vi "PowerSupply.vi"() -> ()   [LabVIEW 2018]
uses:
  classes/Tushars Events Toolkit/Software/Modules/EventClient_ObjectReference.ctl
  classes/Variable Manager/VariableManager_Bool.vi
  Strict Type Controls/Settings Operation.ctl
  ThirdParty/Keithley KE22xx Series/Keithley KE22xx Series.lvlib
  ThirdParty/Agilent E364X Series/Agilent E364X Series.lvlib
  classes/Variable Manager/VariableManager_Double.vi
panel:
  out "Quit":bool
  out "error out":errorcluster
  in  "error in (no error)":errorcluster
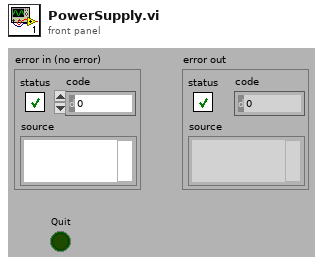
[diagram p1: front panel]
types:
  T1 = cluster{"Port":refnum<visa-resource-name>, "baud rate":u32, "data bits":u16, "parity":enum16{"None", "Odd", "Even", "Mark", "Space"}, "stop bits":u16, "flow control":u16, "timeout":u32}
  T2 = cluster{"PSPort":refnum<visa-resource-name>, "lastUpdate":u32}
  T3 = typedef "EventClient_ObjectReference.ctl" = refnum<k1>
  T4 = typedef "Settings Operation.ctl" = enum8{"Get Value", "Set Value", "Read File", "Write File", "Write Stored Value"}
  T5 = cluster{"Port":refnum<visa-resource-name>, "baud rate":u32, "data bits":u16, "stop bits":u16, "parity":enum16{"None", "Odd", "Even", "Mark", "Space"}, "flow control":u16, "Timeout":u32}
  T6 = cluster{"Instrument Select (Output 1)":string, dbl}
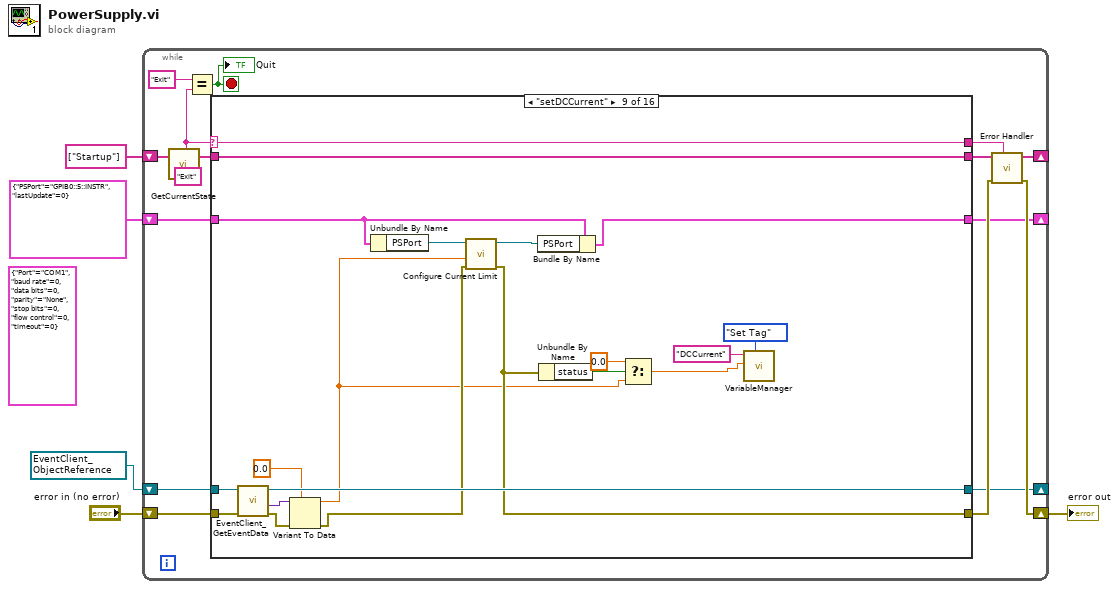
[diagram p0: block diagram]
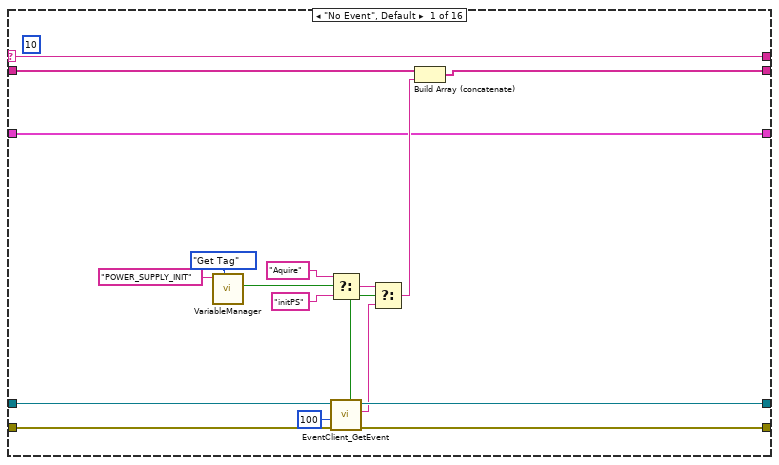
[diagram p2: hidden frame]
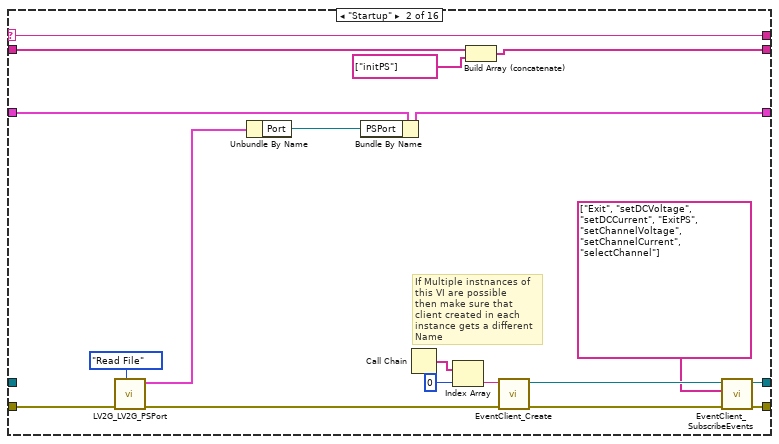
[diagram p3: hidden frame]
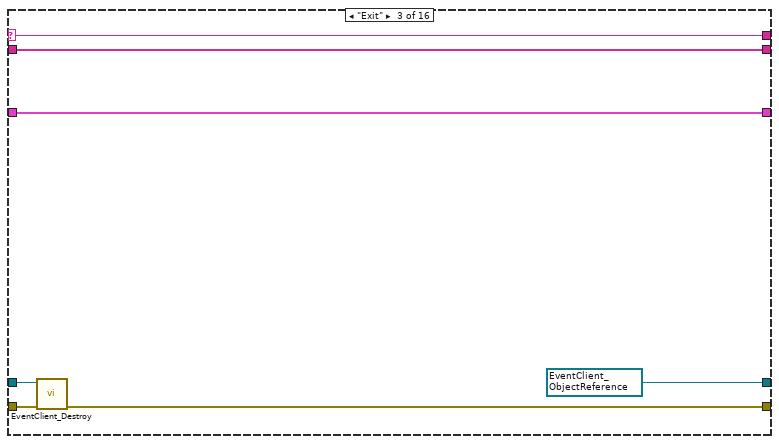
[diagram p4: hidden frame]
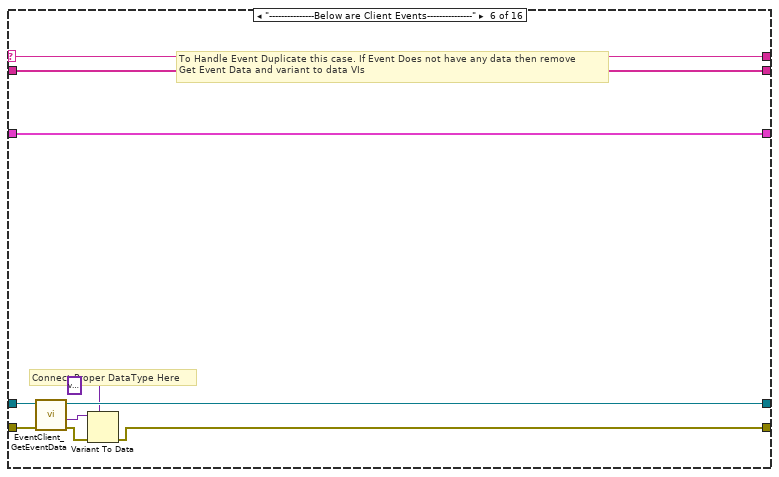
[diagram p7: hidden frame]
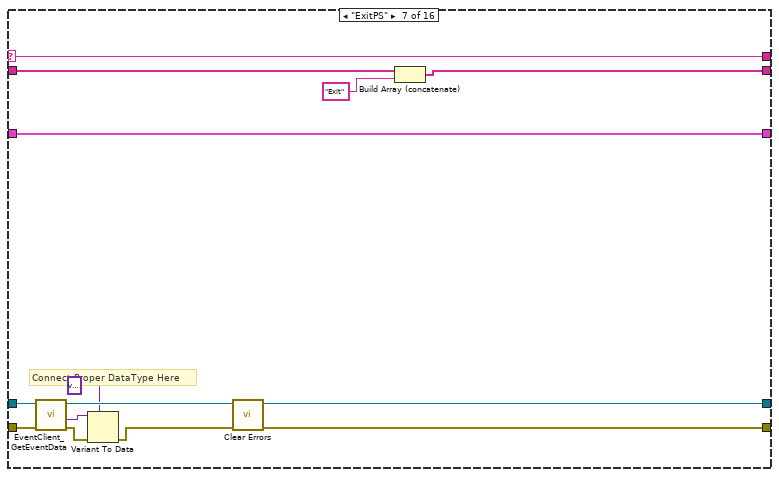
[diagram p8: hidden frame]
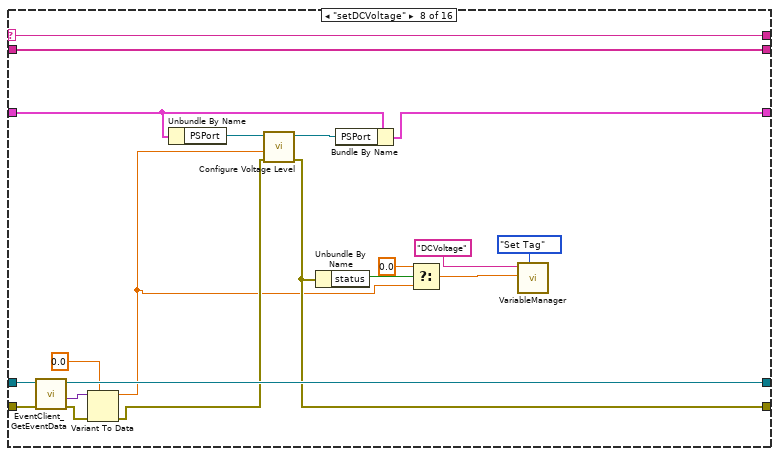
[diagram p9: hidden frame]
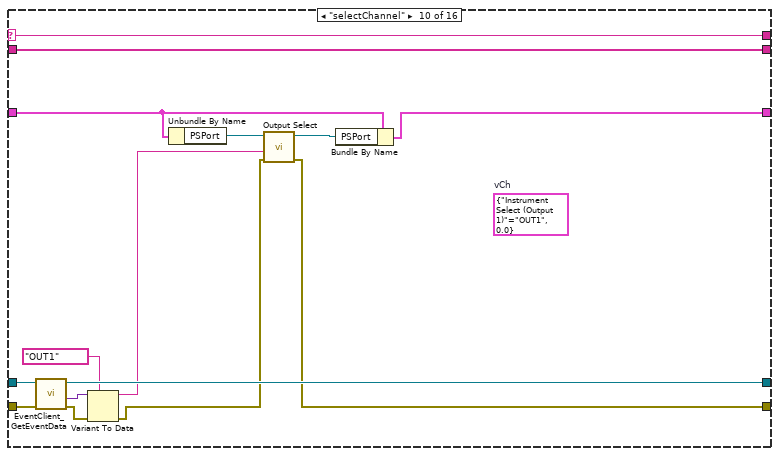
[diagram p10: hidden frame]
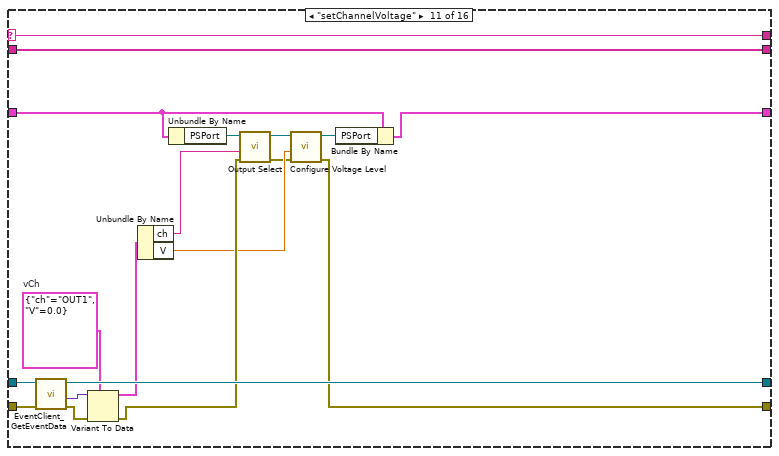
[diagram p11: hidden frame]
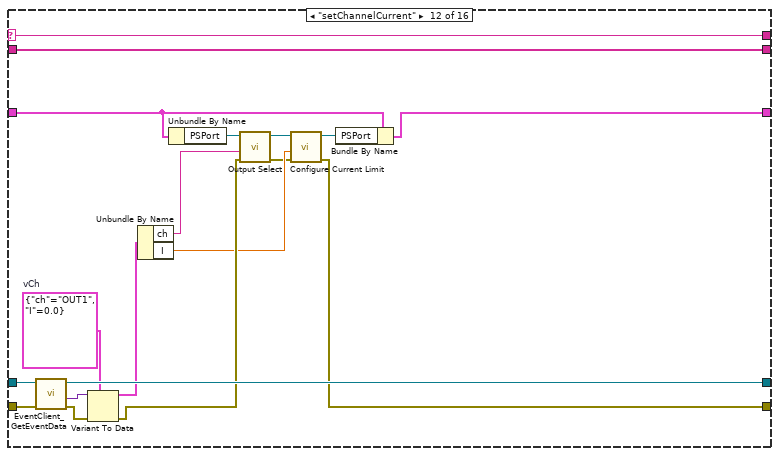
[diagram p12: hidden frame]
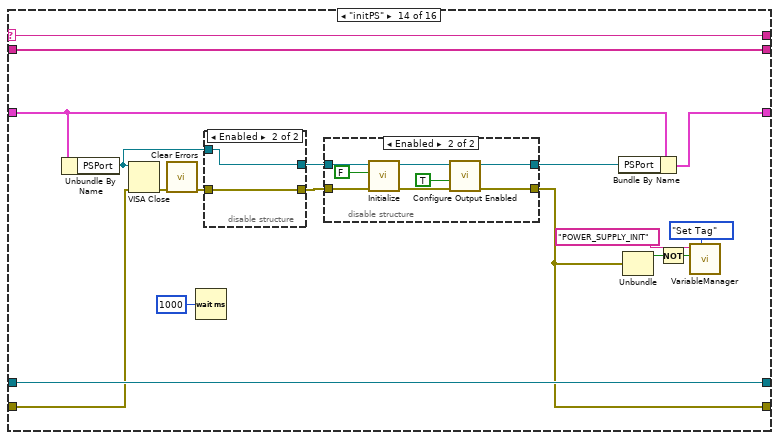
[diagram p14: hidden frame]
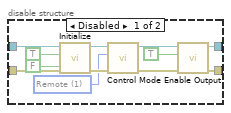
[diagram p15: hidden frame]
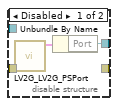
[diagram p16: hidden frame]
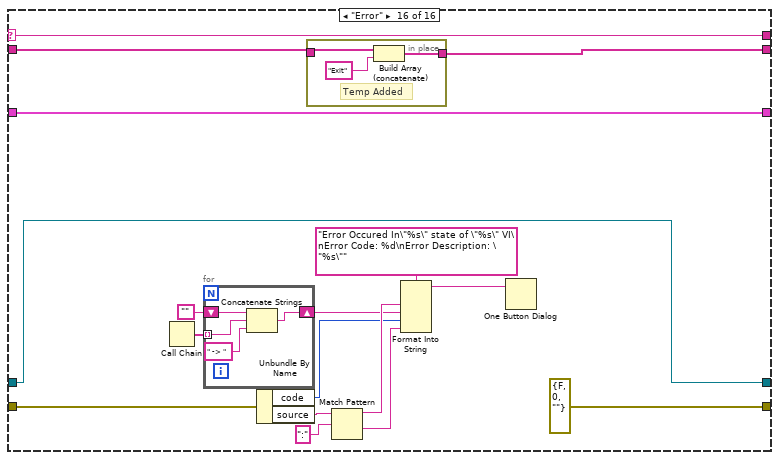
[diagram p18: hidden frame]
diagram:
  (unwired) T1 {"Port"="COM1", "baud rate"=0, "data bits"=0, "parity"=enum."None", "stop bits"=0, "flow control"=0, "timeout"=0} ("Merlin")
  w2 = T3 refnum items=["EventClient"] ("reference")
  n1 = while {
    shift-right: [w16] -> _
    shift-left: string[] ["Startup"] ("State Array Out") -> [w20]
    shift-right: [w12] -> w3
    shift-left: "error in (no error)" -> [w13]
    shift-right: [w9] -> _
    shift-left: w2 -> [w8]
    shift-right: [w6] -> _
    shift-left: T2 {"PSPort"="GPIB0::5::INSTR", "lastUpdate"=0} -> [w7]
    stop <- w17 stop-if-true
    (unwired) "Exit" ("x")
    n2 = call "GetCurrentState.vi"("State Array In"=w20) -> ("Current State"=w10:string, "State Array Out"=w19:string[])  [unwired: 17 in]
    n3 = Equal?(x="Exit", y=w10) -> (x = y?=w17:bool)
    "Quit" <- w17
    n4 = case shown="\"setDCCurrent\"" w10 {
      selector: w10 -> [w38 w57 w64 w68 w73 w83 w96 w116 w136 w151 w170 w189 w194 w212 w243 w260]
      tunnel: w19 -> [w31 w56 w63 w69 w74 w84 w97 w117 w137 w152 w171 w190 w195 w213 w242 w247]
      tunnel: [w33 w55 w63 w69 w74 w84 w88 w117 w137 w152 w171 w190 w195 w213 w242 w244] -> w15
      tunnel: [w35 w49 w60 w67 w72 w79 w85 w103 w122 w141 w153 w172 w193 w199 w241 errorcluster {"status"=FALSE, "code"=0, "source"=""} ("error in (no error)")] -> w11
      tunnel: [w38 w57 w64 w68 w73 w83 w96 w116 w136 w151 w170 w189 w194 w212 w243 w260] -> w14
      tunnel: w13 -> [w36 w44 w61 w67 w72 w81 w94 w114 w134 w149 w168 w187 w193 w197 w241 w248]
      tunnel: [w34 w47 w59 w66 w71 w77 w90 w111 w131 w146 w165 w184 w192 w211 w240 w246] -> w9
      tunnel: w8 -> [w37 _ w62 w66 w71 w82 w95 w115 w135 w150 w169 w188 w192 w211 w240 w246]
      tunnel: w7 -> [w24 w45 w58 w65 w70 w75 w86 w109 w129 w145 w164 w183 w191 w204 w239 w245]
      tunnel: [w24 w40 w58 w65 w70 w75 w86 w108 w128 w144 w163 w182 w191 w203 w239 w245] -> w6
      frame "No Event", Default {
        (unwired) 10
        n5 = call-poly "VariableManager.vi"("Operation"=enum16{"Get Tag", "Set Tag"}."Get Tag", "Tag"="POWER_SUPPLY_INIT") -> ("Value out"=w21:bool)  [unwired: 6 in, 3 out]
        n6 = Select(t="Aquire" ("x"), s=w21, f="initPS" ("x")) -> (s? t:f=w26:string)
        n7 = call "EventClient_GetEvent.vi"("error in (no error)"=w36, "timeout in ms (-1)"=100, "reference"=w37) -> ("error out"=w35:errorcluster, "Name"=w29:string, "reference out"=w34:T3, "timed out?"=w30:bool)  [unwired: 4 in, 1 out]
        n8 = Select(t=w26, s=w30, f=w29) -> (s? t:f=w25:string)
        n9 = Build Array (concatenate)(w31, w25) -> (w33:string[])
      }
      frame "Startup" {
        # "If Multiple instnances of this VI are possible \nthen make sure that client created in each instance gets a different Name"
        n10 = call "LV2G_LV2G_PSPort.vi"("Operation"=Settings_Operation."Read File", "error in (no error)"=w44) -> ("error out"=w43:errorcluster, "Modbus485 Out"=w41:T5)  [unwired: 8 in]
        n11 = Unbundle By Name(w41) -> ("Port"=w39:refnum<visa-resource-name>)
        n12 = Bundle By Name(cluster=w45, "PSPort"=w39) -> (w40:T2)
        n13 = Call Chain() -> (call chain=w53:string[])
        n14 = Index Array(array=w53, index=0) -> (element=w51:string)
        n15 = Build Array (concatenate)(w56, string[] ["initPS"] ("State Array Out")) -> (w55:string[])
        n16 = call "EventClient_Create.vi"("error in (no error)"=w43, "Instance Name"=w51) -> ("error out"=w50:errorcluster, "reference"=w48:T3)  [unwired: 8 in]
        n17 = call "EventClient_SubscribeEvents.vi"("error in (no error)"=w50, "Events"=string[] ["Exit", "setDCVoltage", "setDCCurrent", "ExitPS", "setChannelVoltage", "setChannelCurrent", "selectChannel"], "reference"=w48) -> ("error out"=w49:errorcluster, "reference out"=w47:T3)  [unwired: 7 in]
      }
      frame "Exit" {
        w59 = T3 refnum items=["EventClient"] ("reference out")
        n18 = call "EventClient_Destroy.vi"("error in (no error)"=w61, "reference"=w62) -> ("error out"=w60:errorcluster)  [unwired: 9 in]
      }
      frame "---------------Below are UI Events---------------" {
        # "This State will never Execute\nIt is added just for improving code readability please do not remove this case"
      }
      frame "---------------Below are Menu Events---------------" {
        # "This State will never Execute\nIt is added just for improving code readability please do not remove this case"
      }
      frame "---------------Below are Client Events---------------" {
        # "To Handle Event Duplicate this case. If Event Does not have any data then remove\nGet Event Data and variant to data VIs"
        # "Connect Proper DataType Here"
        n19 = call "EventClient_GetEventData.vi"("error in (no error)"=w81, "reference"=w82) -> ("error out"=w80:errorcluster, "Data"=w78:variant, "reference out"=w77:T3)  [unwired: 7 in]
        n20 = Variant To Data(error in=w80, type=variant, Variant=w78) -> (error out=w79:errorcluster)  [unwired: 1 out]
      }
      frame "ExitPS" {
        # "Connect Proper DataType Here"
        n21 = call "EventClient_GetEventData.vi"("error in (no error)"=w94, "reference"=w95) -> ("error out"=w93:errorcluster, "Data"=w91:variant, "reference out"=w90:T3)  [unwired: 7 in]
        n22 = Variant To Data(error in=w93, type=variant, Variant=w91) -> (error out=w92:errorcluster)  [unwired: 1 out]
        n23 = call <vilib>:"Clear Errors.vi"("error in (no error)"=w92) -> ("error out"=w85:errorcluster)  [unwired: 5 in, 1 out]
        n24 = Build Array (concatenate)(w97, "Exit" ("x")) -> (w88:string[])
      }
      frame "setDCVoltage" {
        n25 = call "EventClient_GetEventData.vi"("error in (no error)"=w114, "reference"=w115) -> ("error out"=w113:errorcluster, "Data"=w112:variant, "reference out"=w111:T3)  [unwired: 7 in]
        n26 = Variant To Data(error in=w113, type=0.0, Variant=w112) -> (data=w100:dbl, error out=w106:errorcluster)
        n27 = Unbundle By Name(w109) -> ("PSPort"=w105:refnum<visa-resource-name>)
        n28 = call "Configure Voltage Level.vi"("error in (no error)"=w106, "Level (0.0 Volts)"=w100, "VISA resource name"=w105) -> ("error out"=w103:errorcluster, "VISA resource name out"=w107:refnum<visa-resource-name>)  [unwired: 7 in]
        n29 = Unbundle By Name(w103) -> ("status"=w101:bool)
        n30 = Bundle By Name(cluster=w109, "PSPort"=w107) -> (w108:T2)
        n31 = Select(t=0.0, s=w101, f=w100) -> (s? t:f=w99:dbl)
        n32 = call-poly "VariableManager.vi"("Operation"=enum16{"Get Tag", "Set Tag"}."Set Tag", "Value"=w99, "Tag"="DCVoltage") -> ()  [unwired: 4 in, 5 out]
      }
      frame "setDCCurrent" {
        n33 = call "EventClient_GetEventData.vi"("error in (no error)"=w134, "reference"=w135) -> ("error out"=w133:errorcluster, "Data"=w132:variant, "reference out"=w131:T3)  [unwired: 7 in]
        n34 = Variant To Data(error in=w133, type=0.0, Variant=w132) -> (data=w120:dbl, error out=w126:errorcluster)
        n35 = Unbundle By Name(w129) -> ("PSPort"=w125:refnum<visa-resource-name>)
        n36 = call "Configure Current Limit.vi"("error in (no error)"=w126, "Current Limit (0.0 Amps)"=w120, "VISA resource name"=w125) -> ("error out"=w122:errorcluster, "VISA resource name out"=w127:refnum<visa-resource-name>)  [unwired: 7 in]
        n37 = Bundle By Name(cluster=w129, "PSPort"=w127) -> (w128:T2)
        n38 = Unbundle By Name(w122) -> ("status"=w121:bool)
        n39 = Select(t=0.0, s=w121, f=w120) -> (s? t:f=w118:dbl)
        n40 = call-poly "VariableManager.vi"("Operation"=enum16{"Get Tag", "Set Tag"}."Set Tag", "Value"=w118, "Tag"="DCCurrent") -> ()  [unwired: 4 in, 5 out]
      }
      frame "selectChannel" {
        (unwired) T6 {"Instrument Select (Output 1)"="OUT1", 0.0}  # vCh
        n41 = call "EventClient_GetEventData.vi"("error in (no error)"=w149, "reference"=w150) -> ("error out"=w148:errorcluster, "Data"=w147:variant, "reference out"=w146:T3)  [unwired: 7 in]
        n42 = Variant To Data(error in=w148, type="OUT1" ("Instrument Select (Output 1)"), Variant=w147) -> (data=w138:string, error out=w142:errorcluster)
        n43 = Unbundle By Name(w145) -> ("PSPort"=w140:refnum<visa-resource-name>)
        n44 = call "Output Select.vi"("error in (no error)"=w142, "Instrument Select (Output 1)"=w138, "VISA resource name"=w140) -> ("error out"=w141:errorcluster, "VISA resource name out"=w143:refnum<visa-resource-name>)  [unwired: 7 in]
        n45 = Bundle By Name(cluster=w145, "PSPort"=w143) -> (w144:T2)
      }
      frame "setChannelVoltage" {
        w158 = cluster{"ch":string, "V":dbl} {"ch"="OUT1", "V"=0.0}  # vCh
        n46 = call "EventClient_GetEventData.vi"("error in (no error)"=w168, "reference"=w169) -> ("error out"=w167:errorcluster, "Data"=w166:variant, "reference out"=w165:T3)  [unwired: 7 in]
        n47 = Variant To Data(error in=w167, type=w158, Variant=w166) -> (data=w159:cluster{"ch":string, "V":dbl}, error out=w161:errorcluster)
        n48 = Unbundle By Name(w159) -> ("ch"=w157:string, "V"=w155:dbl)
        n49 = Unbundle By Name(w164) -> ("PSPort"=w160:refnum<visa-resource-name>)
        n50 = call "Output Select.vi"("error in (no error)"=w161, "Instrument Select (Output 1)"=w157, "VISA resource name"=w160) -> ("error out"=w154:errorcluster, "VISA resource name out"=w162:refnum<visa-resource-name>)  [unwired: 7 in]
        n51 = call "Configure Voltage Level.vi"("error in (no error)"=w154, "Level (0.0 Volts)"=w155, "VISA resource name"=w162) -> ("error out"=w153:errorcluster, "VISA resource name out"=w156:refnum<visa-resource-name>)  [unwired: 7 in]
        n52 = Bundle By Name(cluster=w164, "PSPort"=w156) -> (w163:T2)
      }
      frame "setChannelCurrent" {
        w177 = cluster{"ch":string, "I":dbl} {"ch"="OUT1", "I"=0.0}  # vCh
        n53 = call "EventClient_GetEventData.vi"("error in (no error)"=w187, "reference"=w188) -> ("error out"=w186:errorcluster, "Data"=w185:variant, "reference out"=w184:T3)  [unwired: 7 in]
        n54 = Variant To Data(error in=w186, type=w177, Variant=w185) -> (data=w178:cluster{"ch":string, "I":dbl}, error out=w180:errorcluster)
        n55 = Unbundle By Name(w178) -> ("ch"=w176:string, "I"=w174:dbl)
        n56 = Unbundle By Name(w183) -> ("PSPort"=w179:refnum<visa-resource-name>)
        n57 = call "Output Select.vi"("error in (no error)"=w180, "Instrument Select (Output 1)"=w176, "VISA resource name"=w179) -> ("error out"=w173:errorcluster, "VISA resource name out"=w181:refnum<visa-resource-name>)  [unwired: 7 in]
        n58 = call "Configure Current Limit.vi"("error in (no error)"=w173, "Current Limit (0.0 Amps)"=w174, "VISA resource name"=w181) -> ("error out"=w172:errorcluster, "VISA resource name out"=w175:refnum<visa-resource-name>)  [unwired: 7 in]
        n59 = Bundle By Name(cluster=w183, "PSPort"=w175) -> (w182:T2)
      }
      frame "---------------Below are Subroutine states---------------" {
      }
      frame "initPS" {
        n60 = Unbundle By Name(w204) -> ("PSPort"=w198:refnum<visa-resource-name>)
        n61 = VISA Close(VISA resource name=w198, error in (no error)=w197) -> (error out=w210:errorcluster)
        n62 = call <vilib>:"Clear Errors.vi"("error in (no error)"=w210) -> ("error out"=w205:errorcluster)  [unwired: 5 in, 1 out]
        n63 = Wait (ms)(milliseconds to wait=u32 1000) -> ()  [unwired: 1 out]
        n64 = disable-structure shown="Enabled" {
          disable-tunnel: w205 -> [w235 w237]
          disable-tunnel: [w234 w238] -> w202
          disable-tunnel: w198 -> [_ w238]
          disable-tunnel: [_ w237] -> w196
          frame Disabled {
            n65 = call "LV2G_LV2G_PSPort.vi"("error in (no error)"=w235) -> ("Modbus485 Out"=w236:T5)  [unwired: 9 in, 1 out]
            n66 = Unbundle By Name(w236) -> ("Port"=w234:refnum<visa-resource-name>)
          }
          frame Enabled {
          }
        }
        n67 = disable-structure shown="Enabled" {
          disable-tunnel: w202 -> [w225 w230]
          disable-tunnel: w196 -> [w222 w227]
          disable-tunnel: [w217 w229] -> w200
          disable-tunnel: [w215 w228] -> w199
          frame Disabled {
            w219 = u16 1 items=["Local", "Remote", "Remote Lock"] ("Control Mode (1: Remote)")
            n68 = call "Initialize.vi"("error in (no error)"=w222, "Reset (True)"=FALSE, "ID Query (True)"=TRUE, "VISA resource name"=w225) -> ("error out"=w220:errorcluster, "VISA resource name out"=w221:refnum<visa-resource-name>)  [unwired: 6 in]
            n69 = call "Control Mode.vi"("error in (no error)"=w220, "Control Mode (1: Remote)"=w219, "VISA resource name"=w221) -> ("error out"=w216:errorcluster, "VISA resource name out"=w218:refnum<visa-resource-name>)  [unwired: 7 in]
            n70 = call "Enable Output.vi"("error in (no error)"=w216, "Enable Output (T: Enable)"=TRUE, "VISA resource name"=w218) -> ("error out"=w215:errorcluster, "VISA resource name out"=w217:refnum<visa-resource-name>)  [unwired: 7 in]
          }
          frame Enabled {
            n71 = call "Initialize.vi"("error in (no error)"=w227, "Reset Device (T: Reset)"=FALSE, "VISA resource name"=w230) -> ("error out"=w231:errorcluster, "VISA resource name out"=w233:refnum<visa-resource-name>)  [unwired: 7 in]
            n72 = call "Configure Output Enabled.vi"("error in (no error)"=w231, "Output Enabled (F: Off)"=TRUE, "VISA resource name"=w233) -> ("error out"=w228:errorcluster, "VISA resource name out"=w229:refnum<visa-resource-name>)  [unwired: 7 in]
          }
        }
        n73 = Bundle By Name(cluster=w204, "PSPort"=w200) -> (w203:T2)
        n74 = Unbundle(w199) -> ("status"=w201:bool)  [unwired: 2 out]
        n75 = Not(x=w201) -> (.not. x?=w209:bool)
        n76 = call-poly "VariableManager.vi"("Operation"=enum16{"Get Tag", "Set Tag"}."Set Tag", "Value"=w209, "Tag"="POWER_SUPPLY_INIT") -> ()  [unwired: 5 in, 4 out]
      }
      frame "---------------Below are Error Handling VIs---------------" {
      }
      frame "Error" {
        n77 = Call Chain() -> (call chain=w255:string[])
        n78 = for {
          tunnel: w255 -> [w266] mode=indexing
          shift-right: [w264] -> w252
          shift-left: "" -> [w267]
          n79 = Concatenate Strings(w267, w266, " -> ") -> (w264:string)
        }
        n80 = Unbundle By Name(w248) -> ("code"=w250:i32, "source"=w249:string)
        n81 = in-place {
          in-place-border: w247 -> [w263]
          in-place-border: [w262] -> w244
          # "Temp Added"
          n82 = Build Array (concatenate)(w263, "Exit" ("x")) -> (w262:string[])
        }
        n83 = Match Pattern(string=w249, regular expression=":") -> (before substring=w253:string, after substring=w257:string)  [unwired: 1 in, 2 out]
        n84 = Format Into String(format string="Error Occured In\"%s\" state of \"%s\" VI\nError Code: %d\nError Description: \"%s\"", w253, w252, w250, w257) -> (resulting string=w256:string)  [unwired: 2 in, 1 out]
        n85 = One Button Dialog(message=w256) -> ()  [unwired: 1 in, 1 out]
      }
    }
    n86 = call "Error Handler.vi"("Current State"=w14, "error in (no error)"=w11, "Msg Queue In"=w15) -> ("error out"=w12:errorcluster, "Msg Queue Out"=w16:string[])  [unwired: 7 in]
  }
  "error out" <- w3
